vi "日志、报警信息存储 (子VI).vi"   [LabVIEW 2016, in "超标留样集成.lvlib" / "科盛超标留样.lvlib"]
uses:
  <vilib>/ptbypt/NI_PtbyPt.lvlib
types:
  T1 = cluster{"时间标识":timestamp, "设备":string, "日志信息":string}
  T2 = cluster{"时间标识":timestamp, "设备":string, "日志信息":string, "流程参数":string}
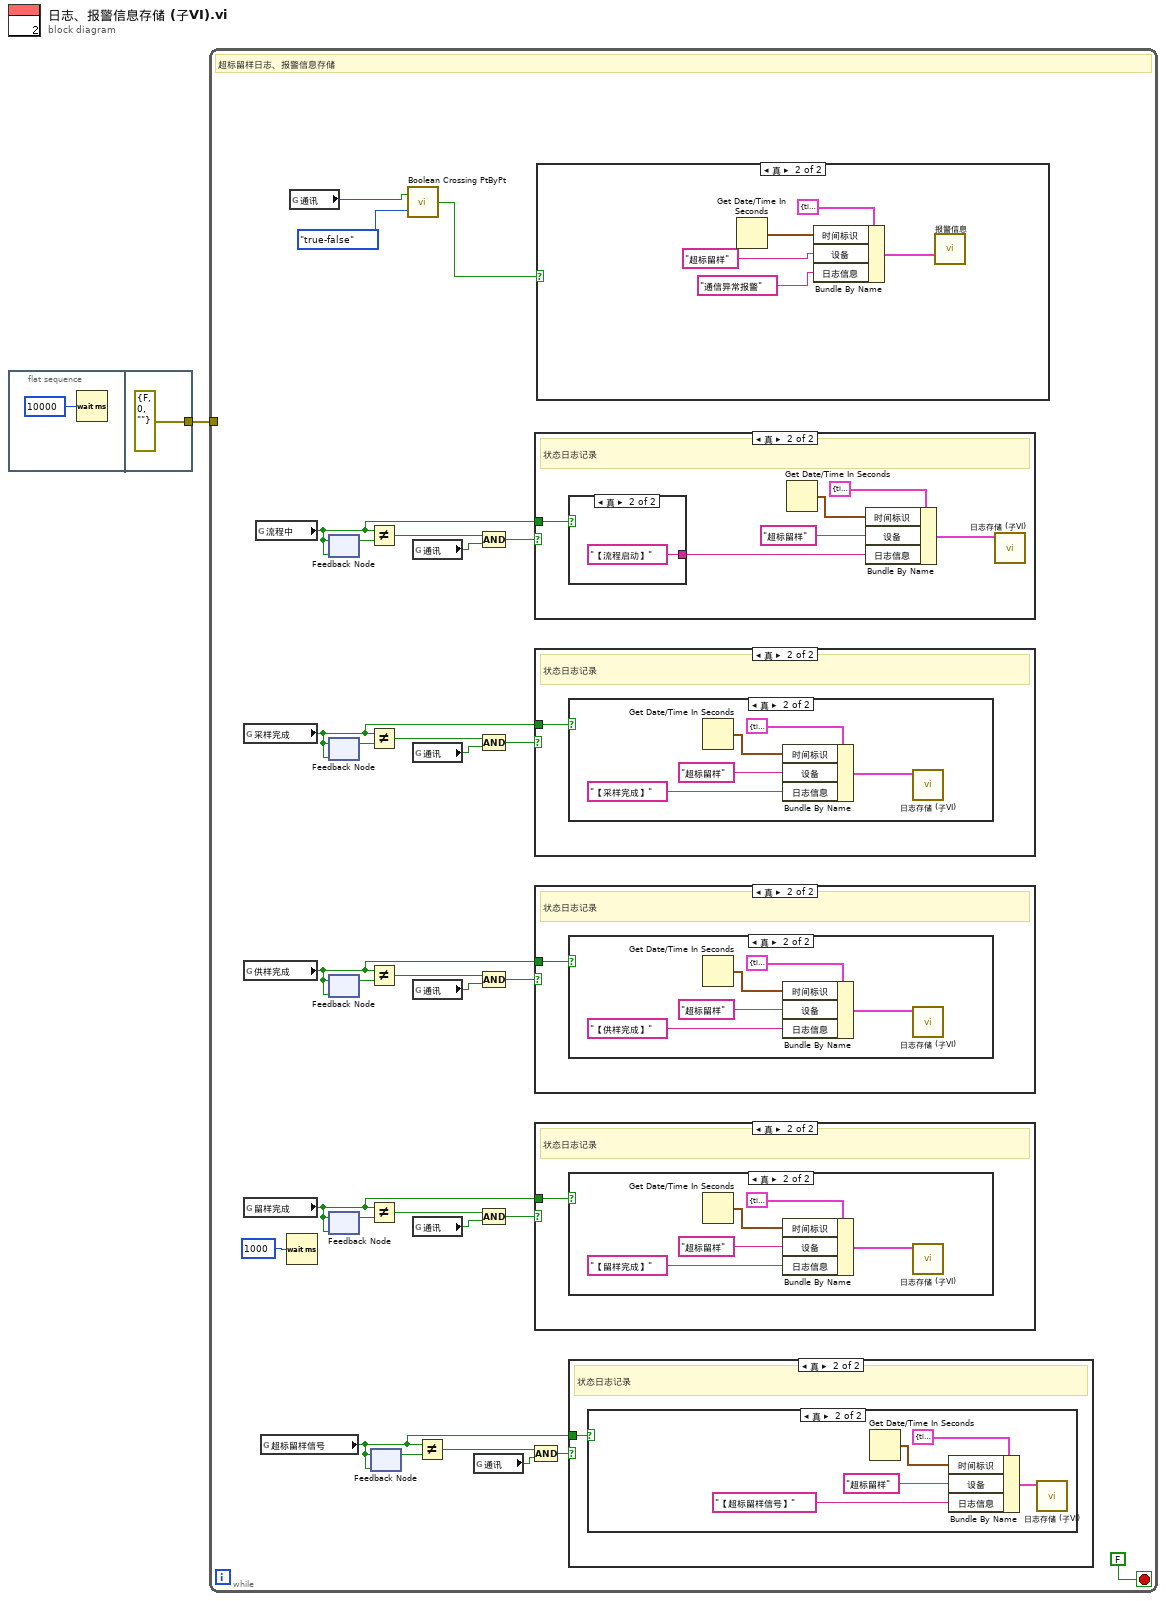
[diagram p0: block diagram]
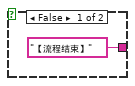
[diagram p12: hidden frame]
diagram:
  n1 = flat-sequence {
    tunnel: [errorcluster {"status"=FALSE, "code"=0, "source"=""} ("错误常量")] -> w1
    frame #0 {
      n2 = Wait (ms)(milliseconds to wait=u32 10000 ("等待时间（毫秒）")) -> ()  [unwired: 1 out]
    }
    frame #1 {
    }
  }
  n3 = while {
    tunnel: w1 -> [_]
    stop <- FALSE stop-if-true
    # "超标留样日志、报警信息存储"
    n4 = global read "超标留样全局.vi" "采样完成"() -> (w23:bool)
    n5 = global read "超标留样全局.vi" "供样完成"() -> (w22:bool)
    n6 = global read "超标留样全局.vi" "留样完成"() -> (w13:bool)
    n7 = global read "超标留样全局.vi" "流程中"() -> (w28:bool)
    n8 = global read "超标留样全局.vi" "超标留样信号"() -> (w8:bool)
    n9 = Wait (ms)(milliseconds to wait=u32 1000 ("等待时间（毫秒）")) -> ()  [unwired: 1 out]
    n10 = global read "超标留样全局.vi" "通讯"() -> (w6:bool)
    n11 = feedback #1(w28) -> (w32:bool)
    n12 = feedback-in #1(w28) -> ()
    n13 = feedback #2(w23) -> (w25:bool)
    n14 = feedback-in #2(w23) -> ()
    n15 = feedback #3(w22) -> (w20:bool)
    n16 = feedback-in #3(w22) -> ()
    n17 = feedback #4(w13) -> (w15:bool)
    n18 = feedback-in #4(w13) -> ()
    n19 = Not Equal?(x=w28, y=w32) -> (x != y?=w31:bool)
    n20 = Not Equal?(x=w23, y=w25) -> (x != y?=w26:bool)
    n21 = Not Equal?(x=w22, y=w20) -> (x != y?=w19:bool)
    n22 = Not Equal?(x=w13, y=w15) -> (x != y?=w16:bool)
    n23 = feedback #5(w8) -> (w11:bool)
    n24 = feedback-in #5(w8) -> ()
    n25 = call <vilib>:"Boolean Crossing PtByPt.vi"("direction"=enum16{"either", "false-true", "true-false"}."true-false", "input"=w6) -> ("crossing"=w4:bool)  [unwired: 1 in]
    n26 = global read "超标留样全局.vi" "通讯"() -> (w30:bool)
    n27 = global read "超标留样全局.vi" "通讯"() -> (w27:bool)
    n28 = global read "超标留样全局.vi" "通讯"() -> (w18:bool)
    n29 = global read "超标留样全局.vi" "通讯"() -> (w17:bool)
    n30 = Not Equal?(x=w8, y=w11) -> (x != y?=w10:bool)
    n31 = global read "超标留样全局.vi" "通讯"() -> (w9:bool)
    n32 = Compound Arithmetic op=AND ("复合运算")(w31, w30) -> (w29:bool)
    n33 = Compound Arithmetic op=AND ("复合运算")(w26, w27) -> (w24:bool)
    n34 = Compound Arithmetic op=AND ("复合运算")(w19, w18) -> (w21:bool)
    n35 = Compound Arithmetic op=AND ("复合运算")(w16, w17) -> (w14:bool)
    n36 = case shown="真" w29 {
      tunnel: w28 -> [_ w64]
      frame False {
      }
      frame True {
        # "状态日志记录"
        n37 = case shown="真" w64 {
          tunnel: ["【流程结束】" ("日志信息") "【流程启动】" ("日志信息")] -> w63
          frame False {
          }
          frame True {
          }
        }
        n38 = Get Date/Time In Seconds() -> (seconds since 1Jan1904=w67:timestamp)
        n39 = Bundle By Name(cluster=T2 {"时间标识"=timestamp(0 s since 1904-01-01), "设备"="", "日志信息"="", "流程参数"=""} ("data in"), "时间标识"=w67, "设备"="超标留样", "日志信息"=w63) -> (w66:T2)
        n40 = call "日志存储 (子VI).vi"("data in"=w66) -> ()  [unwired: 11 in]
      }
    }
    n41 = case shown="真" w24 {
      tunnel: w23 -> [_ w57]
      frame False {
      }
      frame True {
        # "状态日志记录"
        n42 = case shown="真" w57 {
          frame False {
          }
          frame True {
            n43 = Get Date/Time In Seconds() -> (seconds since 1Jan1904=w61:timestamp)
            n44 = Bundle By Name(cluster=T2 {"时间标识"=timestamp(0 s since 1904-01-01), "设备"="", "日志信息"="", "流程参数"=""} ("data in"), "时间标识"=w61, "设备"="超标留样", "日志信息"="【采样完成】") -> (w58:T2)
            n45 = call "日志存储 (子VI).vi"("data in"=w58) -> ()  [unwired: 11 in]
          }
        }
      }
    }
    n46 = case shown="真" w21 {
      tunnel: w22 -> [_ w51]
      frame False {
      }
      frame True {
        # "状态日志记录"
        n47 = case shown="真" w51 {
          frame False {
          }
          frame True {
            n48 = Get Date/Time In Seconds() -> (seconds since 1Jan1904=w55:timestamp)
            n49 = Bundle By Name(cluster=T2 {"时间标识"=timestamp(0 s since 1904-01-01), "设备"="", "日志信息"="", "流程参数"=""} ("data in"), "时间标识"=w55, "设备"="超标留样", "日志信息"="【供样完成】") -> (w52:T2)
            n50 = call "日志存储 (子VI).vi"("data in"=w52) -> ()  [unwired: 11 in]
          }
        }
      }
    }
    n51 = case shown="真" w14 {
      tunnel: w13 -> [_ w45]
      frame False {
      }
      frame True {
        # "状态日志记录"
        n52 = case shown="真" w45 {
          frame False {
          }
          frame True {
            n53 = Get Date/Time In Seconds() -> (seconds since 1Jan1904=w49:timestamp)
            n54 = Bundle By Name(cluster=T2 {"时间标识"=timestamp(0 s since 1904-01-01), "设备"="", "日志信息"="", "流程参数"=""} ("data in"), "时间标识"=w49, "设备"="超标留样", "日志信息"="【留样完成】") -> (w46:T2)
            n55 = call "日志存储 (子VI).vi"("data in"=w46) -> ()  [unwired: 11 in]
          }
        }
      }
    }
    n56 = Compound Arithmetic op=AND ("复合运算")(w10, w9) -> (w12:bool)
    n57 = case shown="真" w4 {
      frame False {
      }
      frame True {
        n58 = Get Date/Time In Seconds() -> (seconds since 1Jan1904=w36:timestamp)
        n59 = Bundle By Name(cluster=T1 {"时间标识"=timestamp(0 s since 1904-01-01), "设备"="", "日志信息"=""} ("data in"), "时间标识"=w36, "设备"="超标留样", "日志信息"="通信异常报警" ("设备")) -> (w37:T1)
        n60 = call "报警信息.vi"("data in"=w37) -> ()  [unwired: 10 in, 1 out]
      }
    }
    n61 = case shown="真" w12 {
      tunnel: w8 -> [_ w39]
      frame False {
      }
      frame True {
        # "状态日志记录"
        n62 = case shown="真" w39 {
          frame False {
          }
          frame True {
            n63 = Get Date/Time In Seconds() -> (seconds since 1Jan1904=w43:timestamp)
            n64 = Bundle By Name(cluster=T2 {"时间标识"=timestamp(0 s since 1904-01-01), "设备"="", "日志信息"="", "流程参数"=""} ("data in"), "时间标识"=w43, "设备"="超标留样", "日志信息"="【超标留样信号】") -> (w40:T2)
            n65 = call "日志存储 (子VI).vi"("data in"=w40) -> ()  [unwired: 11 in]
          }
        }
      }
    }
  }
